vi "Test Target.vi"() -> ()   [LabVIEW 2019]
panel:
  in  "String":string=" 0123"
  in  "Time Stamp":timestamp=timestamp(3600 s since 1904-01-01) format="%^<%x %.3X %Z>T"
  in  "Array of Cluster":T1(array[cluster])=[{"U8"=0, "U16"=0, "U32"=0, "U64"=0, "U8 Array"=[5, 10, 255], "Frequency"=2400000000.0, "DBL Array"=[2400000000.0, 1000.0]}, {"U8"=0, "U16"=0, "U32"=0, "U64"=0, "U8 Array"=[11, 12, 13], "Frequency"=2400000000.0, "DBL Array"=[2400000000.0, 1000.0]}] {"DBL Array" format="%#.3f"; "Frequency" format="%#.3f"}
  in  "Cluster":T2={"U8"=0, "U16"=0, "U32"=0, "U64"=0, "U8 Array"=[5, 10, 255], "Frequency"=2400000000.0, "DBL Array"=[2400000000.0, 1000.0]} {"DBL Array" format="%#.3f"; "Frequency" format="%#.3f"}
  in  "DBL Array":dbl[](array[numeric])=[2400000000.0, 1000.0, 3600.0] format="%#.3f"
  in  "Frequency":dbl=2400000000.0 format="%#.3f"
  in  "U64":u64
  in  "U32":u32
  in  "U16":u16
  in  "U8":u8
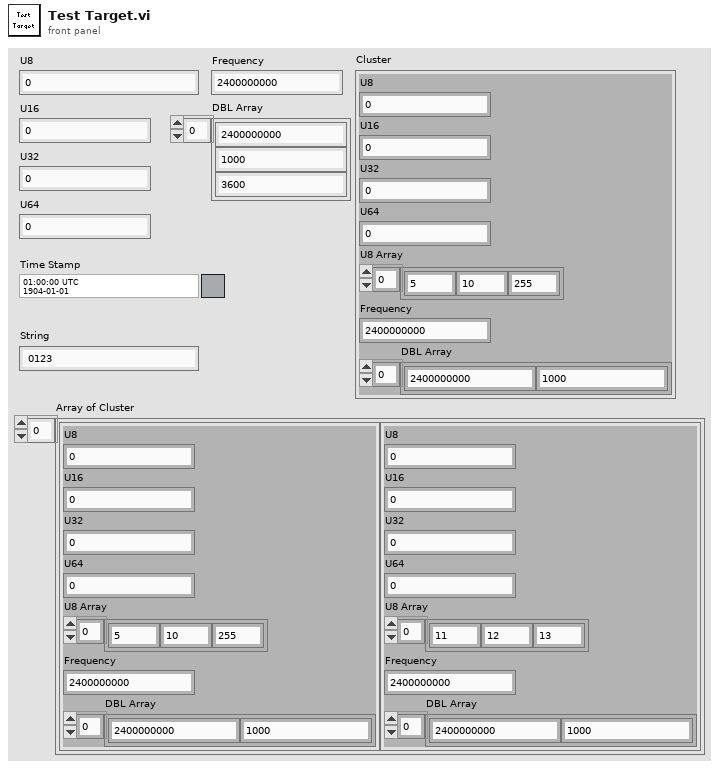
[diagram p1: front panel]
types:
  T1 = cluster{"U8":u8, "U16":u16, "U32":u32, "U64":u64, "U8 Array":u8[], "Frequency":dbl, "DBL Array":dbl[]}[]
  T2 = cluster{"U8":u8, "U16":u16, "U32":u32, "U64":u64, "U8 Array":u8[], "Frequency":dbl, "DBL Array":dbl[]}
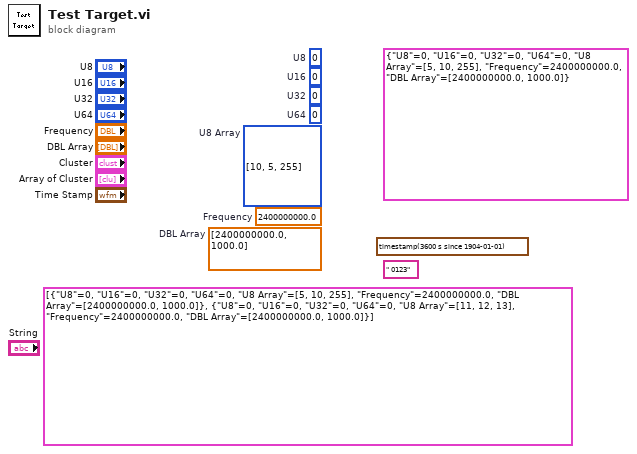
[diagram p0: block diagram]
diagram:
  (unwired) " 0123"
  (unwired) timestamp(3600 s since 1904-01-01) ("Time Stamp")
  (unwired) T1 [{"U8"=0, "U16"=0, "U32"=0, "U64"=0, "U8 Array"=[5, 10, 255], "Frequency"=2400000000.0, "DBL Array"=[2400000000.0, 1000.0]}, {"U8"=0, "U16"=0, "U32"=0, "U64"=0, "U8 Array"=[11, 12, 13], "Frequency"=2400000000.0, "DBL Array"=[2400000000.0, 1000.0]}]
  (unwired) T2 {"U8"=0, "U16"=0, "U32"=0, "U64"=0, "U8 Array"=[5, 10, 255], "Frequency"=2400000000.0, "DBL Array"=[2400000000.0, 1000.0]} ("Cluster")
  (unwired) dbl[] [2400000000.0, 1000.0]  # DBL Array
  (unwired) 2400000000.0  # Frequency
  (unwired) u8[] [10, 5, 255]  # U8 Array
  (unwired) u64 0  # U64
  (unwired) u32 0  # U32
  (unwired) u16 0  # U16
  (unwired) u8 0  # U8
